vi "Calculate Timeout.vi"(4 "error in (no error)":errorcluster, 7 "State Machine Data in":T1 {"Last Sample Time" format="%<%I:%M:%S %p %m/%d>T"}) -> (0 "error out":errorcluster, 3 "State Machine Data out":T1)   [LabVIEW 2015, in "Startup Processes.lvlib"]
uses:
  Startup Processes.lvlib
  _typedefs/State Machine Conditions.ctl
  _typedefs/Machine Modes.ctl
  _typedefs/Subpanel Names.ctl
  Config Data/Config Data.lvclass
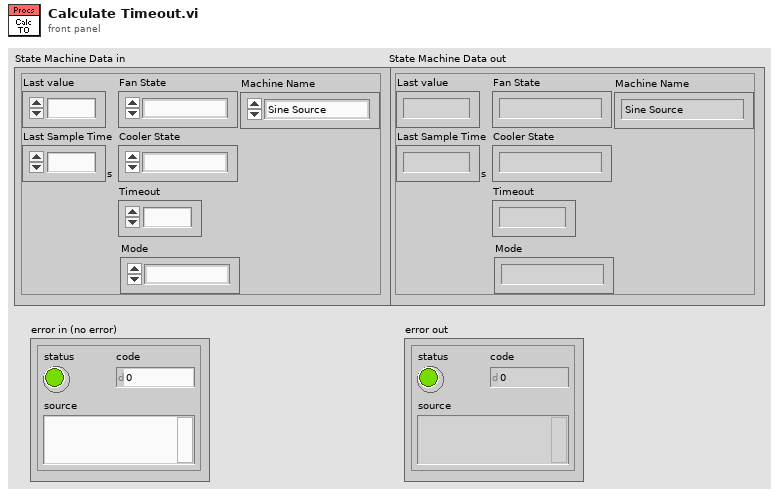
[diagram p1: front panel]
types:
  T1 = typedef "Startup Processes.lvlib/State Machine Conditions.ctl" = cluster{"Last value":dbl, "Last Sample Time":dbl[unit], "Fan State":enum16{"Off", "On"}, "Cooler State":enum16{"Off", "On"}, "Timeout":i32, "Mode":T2, "Machine Name":T3}
  T2 = typedef "Startup Processes.lvlib/Machine Modes.ctl" = enum16{"Startup", "Run"}
  T3 = typedef "Startup Processes.lvlib/Subpanel Names.ctl" = enum16{"Sine Source", "Ramp Source", "Hen House TC", "Dog House TC", "Out House TC"}
  T4 = cluster{"Error High Level":dbl, "Warning High Level":dbl, "Warning Low Level":dbl, "Error Low Level":dbl, "Sample Interval":dbl[unit]}
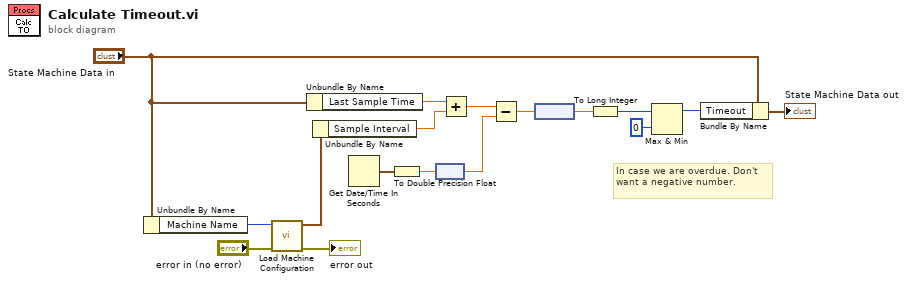
[diagram p0: block diagram]
diagram:
  # "In case we are overdue. Don't want a negative number."
  n1 = Unbundle By Name("State Machine Data in") -> ("Machine Name"=w6:T3)
  n2 = call "Load Machine Configuration.vi"("error in (no error)"="error in (no error)", "Instance Name"=w6) -> ("error out"=→"error out":errorcluster, "TC Parameters"=w5:T4)  [unwired: 4 in]
  n3 = Unbundle By Name("State Machine Data in") -> ("Last Sample Time"=w17:dbl[unit])
  n4 = Unbundle By Name(w5) -> ("Sample Interval"=w4:dbl[unit])
  n5 = Get Date/Time In Seconds() -> (seconds since 1Jan1904=w16:timestamp)
  n6 = To Double Precision Float(number=w16) -> (double precision float=w15:dbl)
  n7 = node(w15) -> (w13:dbl[unit])
  n8 = Add(x=w17, y=w4) -> (x+y=w14:dbl[unit])
  n9 = Subtract(x=w14, y=w13) -> (x-y=w12:dbl[unit])
  n10 = node(w12) -> (w11:dbl)
  n11 = To Long Integer(number=w11) -> (32bit integer=w10:i32)
  n12 = Max & Min(x=w10, y=0) -> (max(x,y)=w8:i32)  [unwired: 1 out]
  n13 = Bundle By Name(cluster="State Machine Data in", "Timeout"=w8) -> (→"State Machine Data out":T1)
